vi "Arm Controller.vi"(8 "error in":errorcluster) -> ()   [LabVIEW 2017]
doc: "This VI executes continuously carrying out the current operation and responding to updates or new operations. It will often contain the timing or control code that is difficult to place directly in TeleOp. This VI generally opens all sensors and motors and isolates the rest of the robot code from knowing how the operations are carried out."
uses:
  <vilib>/Rock Robotics/WPI/Framework/Completion Status.ctl
  Arm Setpoints.ctl
  Arm Operations.ctl
  <vilib>/Rock Robotics/SystemInterfaces/DIO/FPGA_DIOPWMChannel.ctl
  <vilib>/Rock Robotics/SystemInterfaces/DIO/FPGA_DIOChannel.ctl
  <vilib>/Rock Robotics/WPI/Switch/WPI_SwitchOpenLimit.vi
  <vilib>/Rock Robotics/WPI/RobotDrive/WPI_RobotDriveOpen2MotorWithSPARK.vi
  <vilib>/Rock Robotics/Network Tables/NT Write Number.vi
panel:
  out "Switch Value":bool
  in  "Interactive Values":T1
  out "Current\nCmd":string
  in  "Buttons":cluster{"Execute Cmd":bool, "Abort Cmd":bool}
  out "Command Timing":cluster{"Start Time (ms)":u32, "Iterations":i32}
  out "Status":T3
  # "Tip: It may be helpful to observe inputs and sensor values.\nYou may also want to display tuning or debugging controls."
  # "Interactive Command: You may fill in the settings for a command\nand schedule it with the Execute button. You can observe and abort\nany command while fine tuning the code for the controller."
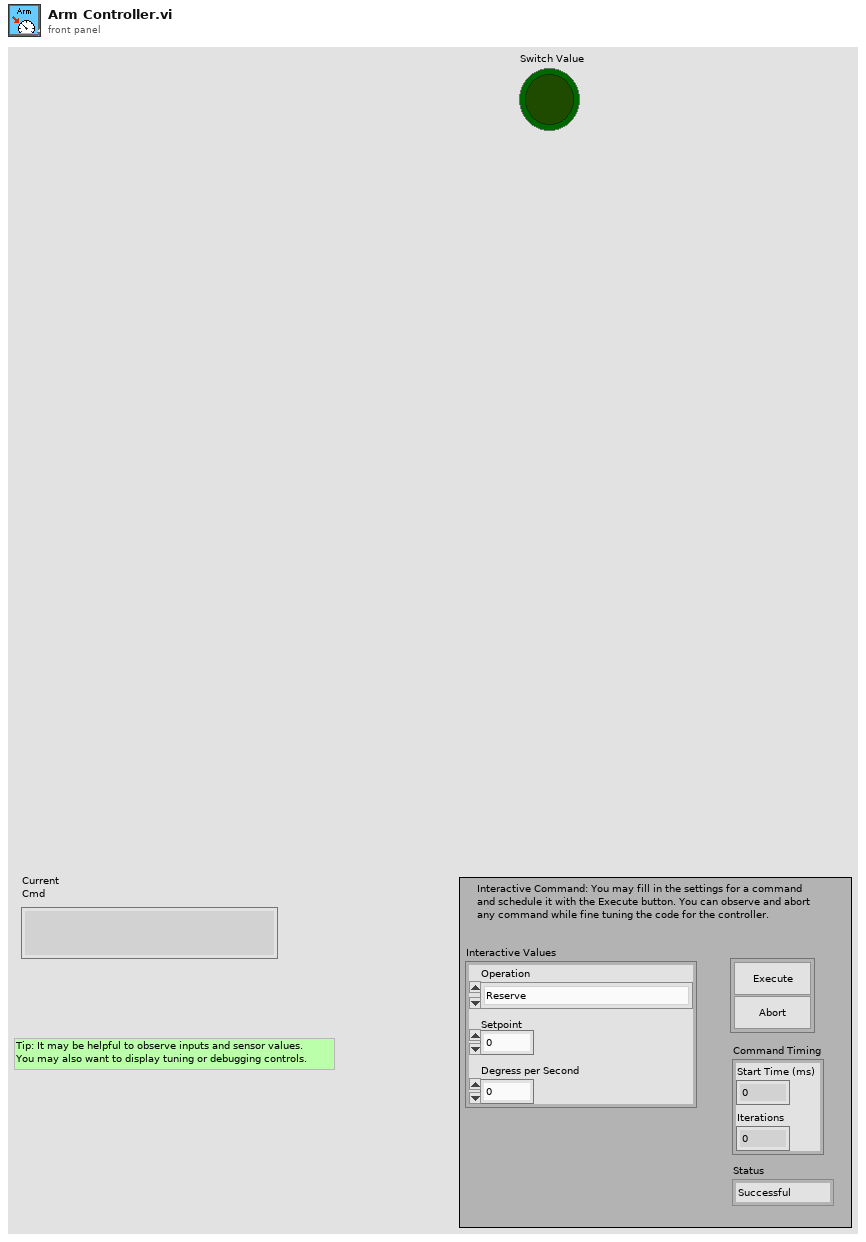
[diagram p1: front panel]
types:
  T1 = typedef "Arm Setpoints.ctl" = cluster{"Operation":T2, "Setpoint":dbl, "Degress per Second":dbl}
  T2 = typedef "Arm Operations.ctl" = enum16{"Reserve", "Read Current", "Immediate", "Lift Arm", "Lower Arm ", "Button Lift Arm", "Button Lower Arm"}
  T3 = typedef "Completion Status.ctl" = enum16{"Successful", "Aborted", "Incomplete"}
  T4 = typedef "FPGA_DIOPWMChannel.ctl" = enum8{"PWM 0", "PWM 1", "PWM 2", "PWM 3", "PWM 4", "PWM 5", "PWM 6", "PWM 7", "PWM 8", "PWM 9", "PWM MXP 0", "PWM MXP 1", "PWM MXP 2", "PWM MXP 3", "PWM MXP 4", "PWM MXP 5", "PWM MXP 6", "PWM MXP 7", "PWM MXP 8", "PWM MXP 9", "Invalid"}
  T5 = typedef "FPGA_DIOChannel.ctl" = enum8{"DIO 0", "DIO 1", "DIO 2", "DIO 3", "DIO 4", "DIO 5", "DIO 6", "DIO 7", "DIO 8", "DIO 9", "DIO MXP 0", "DIO MXP 1", "DIO MXP 2", "DIO MXP 3", "DIO MXP 4", "DIO MXP 5", "DIO MXP 6", "DIO MXP 7", "DIO MXP 8", "DIO MXP 9", "DIO MXP 10", "DIO MXP 11", "DIO MXP 12", "DIO MXP 13", "DIO MXP 14", "DIO MXP 15", "SPI Port CS1", "SPI Port CS2", "SPI Port CS3", "SPI Port MISO", "SPI Port MOSI", "Invalid"}
  T6 = typedef "WPI_RobotDriveDevRef.ctl" = cluster{"DevStatus":errorcluster, "Motors[]":T7[], "Square Inputs":bool, "Max Output":dbl}
  T7 = typedef "WPI_MotorControlDeviceRef.ctl" = cluster{"DeviceStatus":errorcluster, "Type":T8, "PWM":cluster{"PWM Channel":T4, "DeadBand":T9}, "CAN":cluster{"Device Number":u8, "SetOutput VI Ref":variant, "GetOutput VI Ref":variant, "Enable VI Ref":variant, "Disable VI Ref":variant, "Data":variant}, "Invert":bool, "DIO PWM":cluster{"PWM \"Enable\" Channel":T4, "DIOChannel":T5, "PWM Rate":dbl}}
  T8 = typedef "WPI_MotorControlType.ctl" = enum16{"PWM", "CAN", "DIO PWM"}
  T9 = typedef "WPI_PWMDeadband.ctl" = cluster{"Name":string, "maxPositivePwm":i32, "minPositivePwm":i32, "centerPwm":i32, "maxNegativePwm":i32, "minNegativePwm":i32, "angularRange":u16}
  T10 = typedef "WPI_SwitchDevRef.ctl" = cluster{"DevStatus":errorcluster, "DIO Channel":T5, "CntIndex":T11, "Normally Closed":bool}
  T11 = typedef "FPGA_CounterCtrSystemIndex.ctl" = enum8{"Ctr 0", "Ctr 1", "Ctr 2", "Ctr 3", "Ctr 4", "Ctr 5", "Ctr 6", "Ctr 7", "Invalid"}
  T12 = typedef "Command Status Info.ctl" = cluster{"Name":string, "Status":T3, "notifier out":T13}
  T13 = typedef "Completion Notifier.ctl" = refnum<notifier>
  T14 = cluster{"Current Command":T1, "Command Timing":cluster{"Start Time (ms)":u32, "Iterations":i32}, "Command Arguments":cluster{"Command Info":T12, "Description":string, "Default Command":T1, "queue out":refnum<queue>, "Subsystem Name":string}}
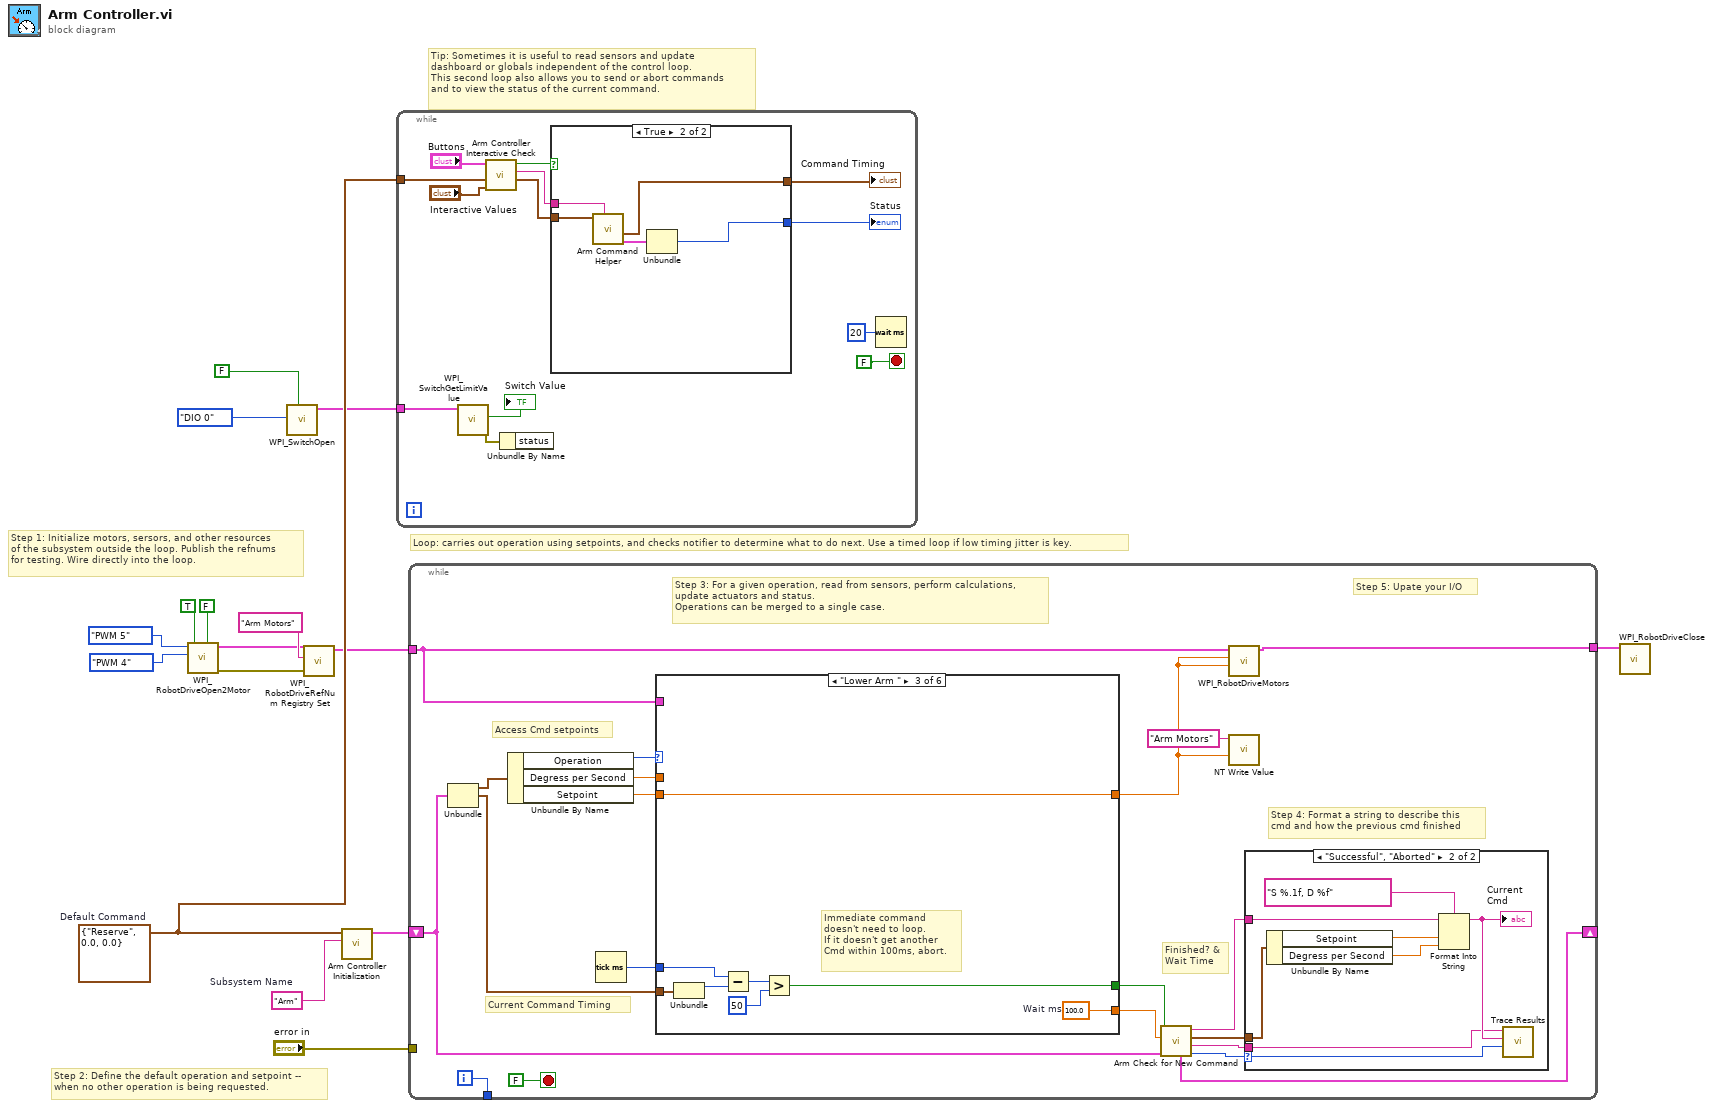
[diagram p0: block diagram]
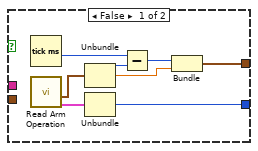
[diagram p2: hidden frame]
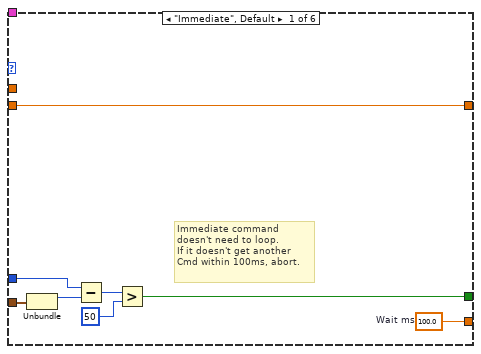
[diagram p4: hidden frame]
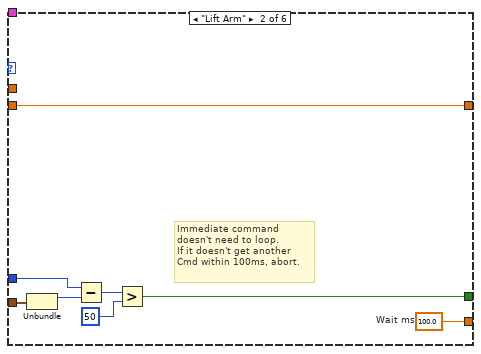
[diagram p5: hidden frame]
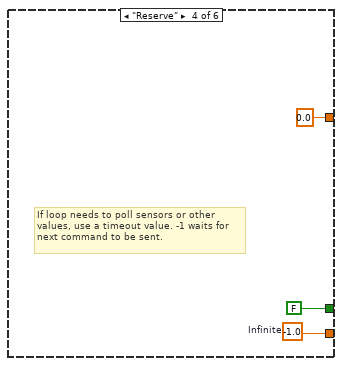
[diagram p6: hidden frame]
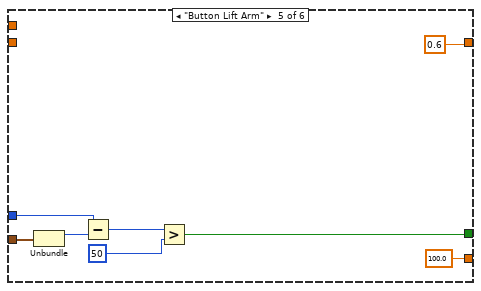
[diagram p7: hidden frame]
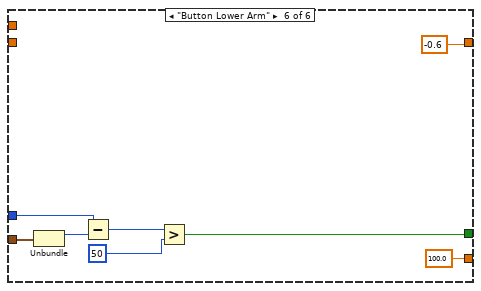
[diagram p8: hidden frame]
diagram:
  w12 = T1 {"Operation"=enum."Reserve", "Setpoint"=0.0, "Degress per Second"=0.0}  # Default Command
  w14 = "Arm"  # Subsystem Name
  # "Tip: Sometimes it is useful to read sensors and update\ndashboard or globals independent of the control loop.\nThis second loop also allows you to send or abort commands\nand to view the status of the current command."
  # "Step 2: Define the default operation and setpoint --\nwhen no other operation is being requested."
  # "Step 1: Initialize motors, sersors, and other resources\nof the subsystem outside the loop. Publish the refnums\nfor testing. Wire directly into the loop."
  # "Loop: carries out operation using setpoints, and checks notifier to determine what to do next. Use a timed loop if low timing jitter is key."
  n1 = call-poly <vilib>:"WPI_RobotDriveOpen2Motor.vi"("Right Motor Inverted"=FALSE, "Left Motor Inverted"=TRUE ("Eliminate Deadband"), "Right Motor"=FPGA_DIOPWMChannel."PWM 4" ("PWM Channel"), "Left Motor"=FPGA_DIOPWMChannel."PWM 5") -> ("error out"=w10:errorcluster, "RobotDriveDevRef"=w2:T6)  [unwired: 6 in]
  n2 = call-poly <vilib>:"WPI_SwitchOpen.vi"("Normally Closed"=FALSE, "DIO Channel"=FPGA_DIOChannel."DIO 0") -> ("SwitchDevRef"=w5:T10)  [unwired: 8 in, 1 out]
  n3 = call <vilib>:"WPI_RobotDriveRefNum Registry Set.vi"("error in (no error)"=w10, "refnum name"="Arm Motors", "RobotDriveDevRef"=w2) -> ("RobotDriveDevRef"=w11:T6)  [unwired: 7 in, 1 out]
  n4 = call "Arm Controller Initialization.vi"("Subsystem Name"=w14, "Default Command"=w12) -> ("Current Command"=w15:T14)  [unwired: 9 in]
  n5 = while {
    tunnel: w12 -> [w26]
    tunnel: w5 -> [w17]
    stop <- FALSE stop-if-true
    n6 = call <vilib>:"WPI_SwitchGetLimitValue.vi"("SwitchDevRef"=w17) -> ("error out"=w18:errorcluster, "Switch Pressed"=→"Switch Value":bool)  [unwired: 8 in, 1 out]
    n7 = call "Arm Controller Interactive Check.vi"("Interactive Command in"="Interactive Values", "Default Command"=w26, "Buttons"="Buttons") -> ("Interactive Command out"=w23:T1, "Trace String"=w24:string, "Schedule"=w25:bool)  [unwired: 6 in]
    n8 = Unbundle By Name(w18) -> ()  [unwired: 1 out]
    n9 = case shown="True" w25 {
      tunnel: [w37 w42] -> w22
      tunnel: w23 -> [_ w40]
      tunnel: [w33 w38] -> w21
      tunnel: w24 -> [_ w41]
      frame False {
        n10 = Tick Count (ms)() -> (millisecond timer value=w32:u32)
        n11 = call "Read Arm Operation.vi"() -> ("Command Info"=w30:T12, "SubSystem Data"=w31:T1)  [unwired: 9 in, 1 out]
        n12 = Unbundle(w31) -> ("Operation"=w36:T2, "Setpoint"=w34:dbl)  [unwired: 1 out]
        n13 = Unbundle(w30) -> ("Status"=w37:T3)  [unwired: 2 out]
        n14 = Subtract(x=w32, y=w36) -> (x-y=w35:u32)
        n15 = Bundle(w35, "Setpoint"=w34) -> (w33:cluster{u32, "Setpoint":dbl})  [unwired: 1 in]
      }
      frame True {
        n16 = call "Arm Command Helper.vi"("Description"=w41, "SubSystem Data"=w40) -> ("Command Info Out"=w39:T12, "Command Timing"=w38:cluster{"Start Time (ms)":u32, "Iterations":i32})  [unwired: 7 in, 1 out]
        n17 = Unbundle(w39) -> ("Status"=w42:T3)  [unwired: 2 out]
      }
    }
    "Status" <- w22
    "Command Timing" <- w21
    n18 = Wait (ms)(milliseconds to wait=u32 20) -> ()  [unwired: 1 out]
  }
  n19 = while {
    shift-right: [w54] -> _
    shift-left: w15 -> [w49]
    tunnel: [w61] -> _
    tunnel: "error in" -> [_]
    tunnel: w11 -> [w45]
    tunnel: [w43] -> w1
    i -> [w61]
    stop <- FALSE stop-if-true
    # "Step 5: Upate your I/O"
    # "Step 4: Format a string to describe this\ncmd and how the previous cmd finished"
    # "Current Command Timing"
    # "Access Cmd setpoints"
    # "Finished? &\nWait Time"
    # "Step 3: For a given operation, read from sensors, perform calculations,\nupdate actuators and status.\nOperations can be merged to a single case."
    n20 = Unbundle(w49) -> ("Current Command"=w60:T1, "Command Timing"=w56:cluster{"Start Time (ms)":u32, "Iterations":i32})  [unwired: 1 out]
    n21 = Unbundle By Name(w60) -> ("Operation"=w59:T2, "Degress per Second"=w58:dbl, "Setpoint"=w55:dbl)
    n22 = Tick Count (ms)() -> (millisecond timer value=w57:u32)
    n23 = case shown="\"Lower Arm \"" w59 {
      tunnel: [w78 w86 w94 w97 100.0 ("Infinite") 100.0 ("Infinite")] -> w47
      tunnel: [w72 w80 w88 FALSE ("ignore previous (F)") w99 w107] -> w48
      tunnel: w56 -> [w74 w82 w90 _ w104 w112]
      tunnel: w58 -> [_ _ _ _ _ _]
      tunnel: w57 -> [w73 w81 w89 _ w105 w113]
      tunnel: w55 -> [w71 w79 w87 _ _ _]
      tunnel: [w71 w79 w87 0.0 ("Angle") 0.6 ("Output") -0.6 ("Output")] -> w44
      tunnel: w45 -> [_ _ _ _ _ _]
      frame "Immediate", Default {
        w78 = 100.0  # Wait ms
        # "Immediate command\ndoesn't need to loop.\nIf it doesn't get another\nCmd within 100ms, abort."
        n24 = Unbundle(w74) -> ("Start Time (ms)"=w77:u32)  [unwired: 1 out]
        n25 = Subtract(x=w73, y=w77) -> (x-y=w76:u32)
        n26 = Greater?(x=w76, y=u8 50 ("Left Motor")) -> (0:w72:bool)
      }
      frame "Lift Arm" {
        w86 = 100.0  # Wait ms
        # "Immediate command\ndoesn't need to loop.\nIf it doesn't get another\nCmd within 100ms, abort."
        n27 = Unbundle(w82) -> ("Start Time (ms)"=w85:u32)  [unwired: 1 out]
        n28 = Subtract(x=w81, y=w85) -> (x-y=w84:u32)
        n29 = Greater?(x=w84, y=u8 50 ("Left Motor")) -> (0:w80:bool)
      }
      frame "Lower Arm " {
        w94 = 100.0  # Wait ms
        # "Immediate command\ndoesn't need to loop.\nIf it doesn't get another\nCmd within 100ms, abort."
        n30 = Unbundle(w90) -> ("Start Time (ms)"=w93:u32)  [unwired: 1 out]
        n31 = Subtract(x=w89, y=w93) -> (x-y=w92:u32)
        n32 = Greater?(x=w92, y=u8 50 ("Left Motor")) -> (0:w88:bool)
      }
      frame "Reserve" {
        w97 = -1.0  # Infinite
        # "If loop needs to poll sensors or other\nvalues, use a timeout value. -1 waits for\nnext command to be sent."
      }
      frame "Button Lift Arm" {
        n33 = Unbundle(w104) -> ("Start Time (ms)"=w103:u32)  [unwired: 1 out]
        n34 = Subtract(x=w105, y=w103) -> (x-y=w102:u32)
        n35 = Greater?(x=w102, y=u8 50 ("Left Motor")) -> (0:w99:bool)
      }
      frame "Button Lower Arm" {
        n36 = Unbundle(w112) -> ("Start Time (ms)"=w111:u32)  [unwired: 1 out]
        n37 = Subtract(x=w113, y=w111) -> (x-y=w110:u32)
        n38 = Greater?(x=w110, y=u8 50 ("Left Motor")) -> (0:w107:bool)
      }
    }
    n39 = call "Arm Check for New Command.vi"("Current Command"=w49, "Wait time (ms)"=w47, "Finished?"=w48) -> ("Completion"=w50:T3, "Subsystem Name"=w51:string, "Current Command"=w52:T1, "Initial Trace String"=w53:string, "NextCommand"=w54:T14)  [unwired: 4 in]
    n40 = call <vilib>:"WPI_RobotDriveMotors.vi"("RightSpeed"=w44, "LeftSpeed"=w44, "RobotDriveDevRef"=w45) -> ("RobotDriveDevRef"=w43:T6)  [unwired: 6 in, 2 out]
    n41 = call-poly <vilib>:"NT Write Value.vi"("Numeric"=w44, "Name"="Arm Motors") -> ()  [unwired: 9 in, 1 out]
    n42 = case shown="\"Successful\", \"Aborted\"" w50 {
      selector: w50 -> [_ w70]
      tunnel: w53 -> [_ w66]
      tunnel: w52 -> [_ w67]
      tunnel: w51 -> [_ w63]
      frame "Incomplete", Default {
        # "Continuing current command"
      }
      frame "Successful", "Aborted" {
        # "Report and setup for next command"
        n43 = Unbundle By Name(w67) -> ("Setpoint"=w69:dbl, "Degress per Second"=w64:dbl)
        n44 = Format Into String(format string="S %.1f, D %f", initial string=w66, w69, w64) -> (resulting string=w65:string)  [unwired: 1 in, 1 out]
        "Current\nCmd" <- w65
        n45 = call <vilib>:"Trace Results.vi"("Status of previous command"=w70, "Description"=w65, "Subsystem"=w63) -> ()  [unwired: 9 in]
      }
    }
  }
  n46 = call <vilib>:"WPI_RobotDriveClose.vi"("RobotDriveDevRef"=w1) -> ()  [unwired: 10 in, 1 out]
